vi "Extract Contour Features.vi"(8 "error in (no error)":errorcluster, 10 "ROI Descriptor":T2 {"Contours"."Type" items=["No Selection", "Point", "Line", "Rectangle", "Oval", "Polygon", "Freehand Region", "Annulus", "Unused2", "Unused3", "Broken Line", "Freehand Line", "Rotated Rectangle"]}, 11 "Image":T1) -> (0 "error out":errorcluster, 1 "Contours Extracted?":bool, 2 "Contour Features":dbl[](array[numeric]), 3 "Image Out":T1)   [LabVIEW 2013]
uses:
  <vilib>/vision/Image Controls.llb/IMAQ Image.ctl
  <vilib>/vision/Contour.llb/IMAQ Contour Curve Extraction.ctl
  <vilib>/vision/NI_Vision_Development_Module.lvlib
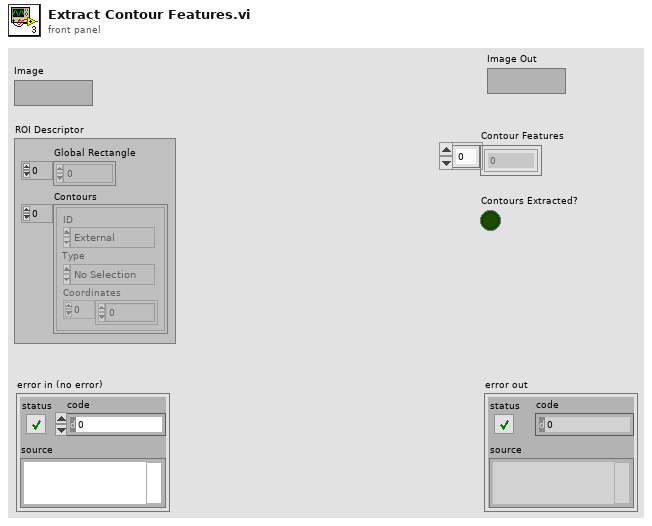
[diagram p1: front panel]
types:
  T1 = typedef "IMAQ Image.ctl" = refnum<image>
  T2 = typedef "ROI Descriptor" = cluster{"Global Rectangle":i32[], "Contours":cluster{"ID":enum32{"External", "Internal"}, "Type":u32, "Coordinates":i32[]}[]}
  T3 = typedef "IMAQ Contour Curve Extraction.ctl" = cluster{"Extraction Mode":u32, "Edge Threshold":i32, "Edge Filter Size":u32, "Min Length":i32, "Search Step Size":i32, "Max Endpoint Gap":i32, "Subpixel":bool}
  T4 = enum16{"Rect Left To Right", "Rect Right To Left", "Rect Top To Bottom", "Rect Bottom To Top", "Annulus Inner To Outer", "Annulus Outer To Inner", "Annulus Start Angle To End Angle", "Annulus End Angle To Start Angle"}
  T5 = enum16{"Closest To Search Start", "Maximum Length", "Strongest Mean Gradient Change"}
  T6 = cluster{"Overlay?":bool, "Color":u32, "Width":u32, "Maintain Width?":bool}
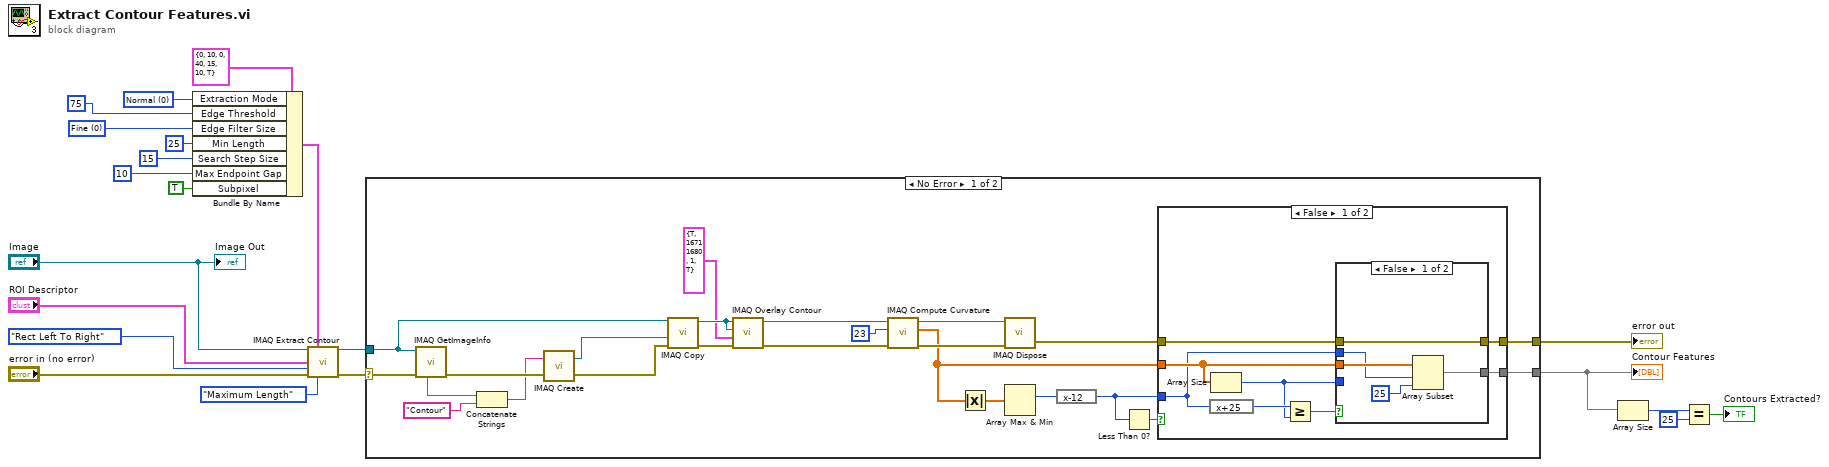
[diagram p0: block diagram]
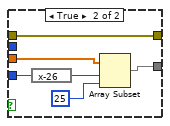
[diagram p2: hidden frame]
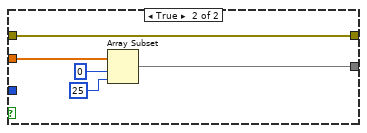
[diagram p3: hidden frame]
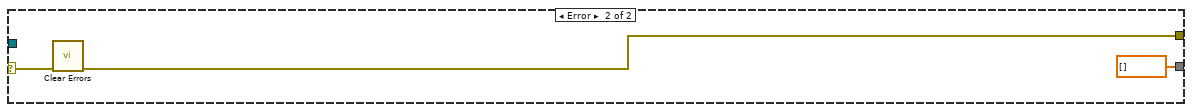
[diagram p4: hidden frame]
diagram:
  w9 = u32 0 items=["Fine", "Normal", "Contour Tracing"] ("Edge Filter Size")
  w14 = u32 0 items=["Normal", "Uniform Regions"] ("Extraction Mode")
  n1 = Bundle By Name(cluster=T3 {"Extraction Mode"=0, "Edge Threshold"=10, "Edge Filter Size"=0, "Min Length"=40, "Search Step Size"=15, "Max Endpoint Gap"=10, "Subpixel"=TRUE} ("Curve Extraction"), "Extraction Mode"=w14, "Edge Threshold"=75, "Edge Filter Size"=w9, "Min Length"=25, "Search Step Size"=15, "Max Endpoint Gap"=10, "Subpixel"=TRUE) -> (w15:T3)
  n2 = call "IMAQ Extract Contour"("Source Image"="Image", "Curve Extraction"=w15, "ROI Descriptor"="ROI Descriptor", "Search Direction"=T4."Rect Left To Right", "error in (no error)"="error in (no error)", "Contour Selection"=T5."Maximum Length") -> ("Source Image Out"=w6:T1, "error out"=w7:errorcluster)  [unwired: 2 in, 6 out]
  n3 = case shown="No Error" w7 {
    selector: w7 -> [w32 w72]
    tunnel: w6 -> [w31 _]
    tunnel: [w23 w71] -> w5
    tunnel: [w22 dbl[] []] -> w4
    frame No Error {
      n4 = call "IMAQ GetImageInfo"("error in (no error)"=w32, "Image"=w31) -> ("error out"=w37:errorcluster, "Image Name"=w39:string)  [unwired: 2 in, 6 out]
      n5 = Concatenate Strings(w39, "Contour" ("string")) -> (w36:string)
      n6 = call "IMAQ Create"("Image Name"=w36, "error in (no error)"=w37) -> ("New Image"=w34:T1, "error out"=w35:errorcluster)  [unwired: 3 in]
      n7 = call "IMAQ Copy"("error in (no error)"=w35, "Image Dst"=w34, "Image Src"=w31) -> ("error out"=w45:errorcluster, "Image Dst Out"=w44:T1)  [unwired: 3 in]
      n8 = call "IMAQ Overlay Contour"("error in (no error)"=w45, "Contour Points Settings"=T6 {"Overlay?"=TRUE, "Color"=16711680, "Width"=1, "Maintain Width?"=TRUE}, "Contour Image"=w44, "Image"=w44) -> ("error out"=w42:errorcluster, "Image Out"=w41:T1)  [unwired: 2 in, 4 out]
      n9 = call "IMAQ Compute Curvature"("error in (no error)"=w42, "Kernel Width"=u32 23, "Contour Image"=w41) -> ("error out"=w30:errorcluster, "Curvature Profile (pixel)"=w25:dbl[], "Contour Image Out (dup)"=w29:T1)  [unwired: 1 in, 5 out]
      n10 = Absolute Value(x=w25) -> (abs(x)=w33:dbl[])
      n11 = call "IMAQ Dispose"("Image"=w29, "error in (no error)"=w30) -> ("error out"=w24:errorcluster)  [unwired: 4 in]
      n12 = Array Max & Min(array=w33) -> (max index (indices)=w28:i32)  [unwired: 3 out]
      n13 = expression code="x-12"(w28) -> (w27:i32)
      n14 = Less Than 0?(x=w27) -> (x < 0?=w26:bool)
      n15 = case shown="False" w26 {
        tunnel: w27 -> [w46 _]
        tunnel: w25 -> [w51 w69]
        tunnel: [w48 w66] -> w22
        tunnel: w24 -> [w50 w65]
        tunnel: [w47 w65] -> w23
        frame False {
          n16 = expression code="x+25"(w46) -> (w53:i32)
          n17 = Array Size(array=w51) -> (size(s)=w49:i32)
          n18 = Greater Or Equal?(x=w53, y=w49) -> (x >= y?=w52:bool)
          n19 = case shown="False" w52 {
            tunnel: w51 -> [w58 w61]
            tunnel: w50 -> [w56 w59]
            tunnel: w49 -> [_ w64]
            tunnel: [w57 w60] -> w48
            tunnel: [w56 w59] -> w47
            tunnel: w46 -> [w55 _]
            frame False {
              n20 = Array Subset(array=w58, index=w55, length=25) -> (w57:dbl[])
            }
            frame True {
              n21 = expression code="x-26"(w64) -> (w63:i32)
              n22 = Array Subset(array=w61, index=w63, length=25) -> (w60:dbl[])
            }
          }
        }
        frame True {
          n23 = Array Subset(array=w69, index=0, length=25) -> (w66:dbl[])
        }
      }
    }
    frame Error {
      n24 = call <vilib>:"Clear Errors.vi"("error in (no error)"=w72) -> ("error out"=w71:errorcluster)  [unwired: 6 in]
    }
  }
  "error out" <- w5
  "Contour Features" <- w4
  n25 = Array Size(array=w4) -> (size(s)=w2:i32)
  n26 = Equal?(x=w2, y=25) -> (x = y?=→"Contours Extracted?":bool)
  "Image Out" <- "Image"
